vi "init_AO_task.vi"(5 "new task name":string="QScope AO-task", 8 "error in":errorcluster, 9 "samples per channel":i32=1000, 10 "rate":dbl=1000.0 format="%0.2f", 11 "AO channel list":string[](array[string])) -> (0 "error out":errorcluster, 3 "task out":refnum<k21>)   [LabVIEW 2018]
uses:
  <vilib>/DAQmx/create/channels.llb/DAQmx Create Channel (AO-Voltage-Basic).vi
  <vilib>/DAQmx/configure/timing.llb/DAQmx Timing (Sample Clock).vi
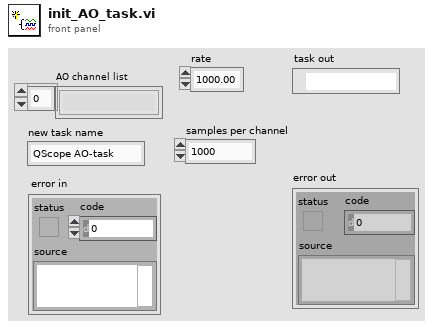
[diagram p1: front panel]
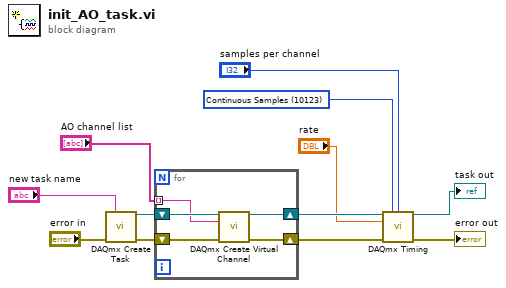
[diagram p0: block diagram]
diagram:
  w4 = 10123 items=["Finite Samples"=10178, "Continuous Samples"=10123, "Hardware Timed Single Point"=12522] ("sample mode")
  n1 = call <vilib>:"DAQmx Create Task.vi"("new task name"="new task name", "error in"="error in") -> ("task out"=w12:refnum<k21>, "error out"=w11:errorcluster)  [unwired: 12 in]
  n2 = for {
    tunnel: "AO channel list" -> [w15] mode=indexing
    shift-right: [w14] -> w7
    shift-left: w12 -> [w17]
    shift-right: [w13] -> w6
    shift-left: w11 -> [w16]
    n3 = call-poly <vilib>:"DAQmx Create Virtual Channel.vi"("task in"=w17, "physical channels"=w15, "error in"=w16) -> ("task out"=w14:refnum<k21>, "error out"=w13:errorcluster)  [unwired: 11 in]
  }
  n4 = call-poly <vilib>:"DAQmx Timing.vi"("task/channels in"=w7, "sample mode"=w4, "samples per channel"="samples per channel", "rate"="rate", "error in"=w6) -> ("task out"=→"task out":refnum<k21>, "error out"=→"error out":errorcluster)  [unwired: 9 in]
